vi "Magnet_Initialize.vi"(8 "error in (no error)":errorcluster) -> (0 "error out":errorcluster, 3 "VISA resource name out":refnum<visa-resource-name>)   [LabVIEW 2010]
uses:
  <instrlib>/Keithley 24XX/Keithley 24XX.lvlib
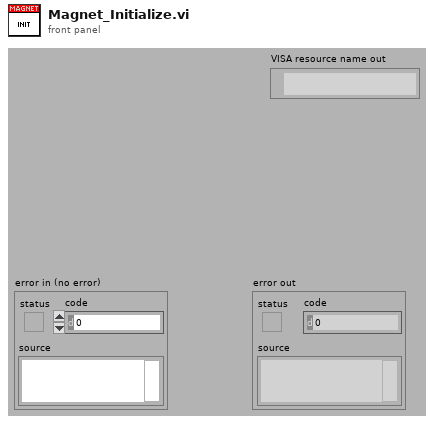
[diagram p1: front panel]
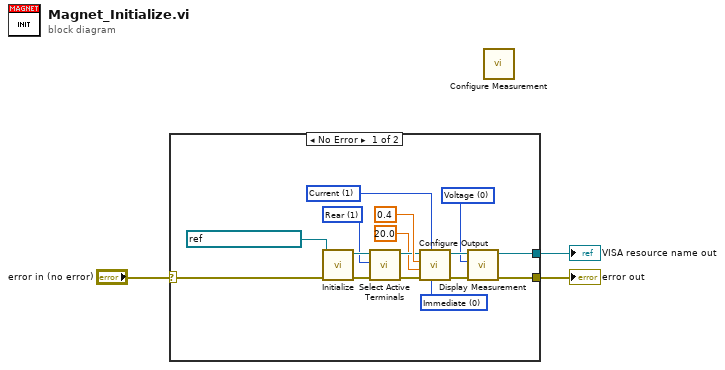
[diagram p0: block diagram]
diagram:
  n1 = case shown="No Error" "error in (no error)" {
    selector: "error in (no error)" -> [w7 w20]
    tunnel: [w4 w20] -> w2
    tunnel: [w5 _] -> w1
    frame No Error {
      w8 = u16 0 items=["Immediate", "Triggered"] ("Output Type  (0: Immediate)")
      w9 = u16 0 items=["Voltage", "Current", "Resistance"] ("Displayed Measurement (0: Voltage)")
      w12 = u16 1 items=["Voltage", "Current"] ("Source Mode  (0: Voltage)")
      w17 = u16 1 items=["Front", "Rear"] ("Active Terminals (0: Front)")
      n2 = call <instrlib>:"Initialize.vi"("error in (no error)"=w7, "VISA resource name"=refnum<visa-resource-name> "GPIB0::10::INSTR") -> ("error out"=w19:errorcluster, "VISA resource name out"=w18:refnum<visa-resource-name>)  [unwired: 8 in]
      n3 = call <instrlib>:"Select Active Terminals.vi"("error in (no error)"=w19, "Active Terminals (0: Front)"=w17, "VISA resource name"=w18) -> ("error out"=w14:errorcluster, "VISA resource name out"=w15:refnum<visa-resource-name>)  [unwired: 7 in]
      n4 = call <instrlib>:"Configure Output.vi"("Output Type  (0: Immediate)"=w8, "Source Mode  (0: Voltage)"=w12, "error in (no error)"=w14, "Compliance  Level (0.1)"=20.0, "Output Level (0)"=0.4, "VISA resource name"=w15) -> ("error out"=w11:errorcluster, "VISA resource name out"=w10:refnum<visa-resource-name>)  [unwired: 4 in]
      n5 = call <instrlib>:"Display Measurement.vi"("error in (no error)"=w11, "Displayed Measurement (0: Voltage)"=w9, "VISA resource name"=w10) -> ("error out"=w4:errorcluster, "VISA resource name out"=w5:refnum<visa-resource-name>)  [unwired: 7 in]
    }
    frame Error {
    }
  }
  "error out" <- w2
  "VISA resource name out" <- w1
  n6 = call <instrlib>:"Configure Measurement.vi"() -> ()  [unwired: 10 in, 2 out]
